vi "OpenDataLogFileForReading.vi"(0 "Filename":string) -> (1 "Data Log File Refnum":refnum<k1>, 2 "error out":errorcluster)   [LabVIEW 2010]
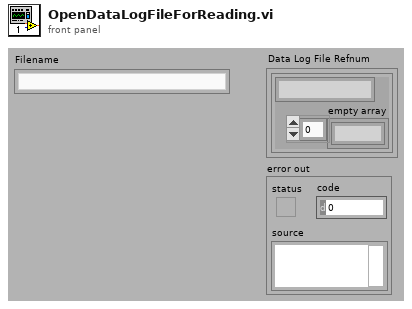
[diagram p1: front panel]
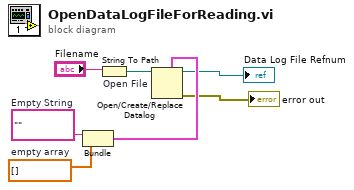
[diagram p0: block diagram]
diagram:
  w7 = ""  # Empty String
  w6 = sgl[] []  # empty array
  n1 = Bundle(w7, "empty array"=w6) -> (w3:cluster{string, "empty array":sgl[]})  [unwired: 1 out]
  n2 = String To Path(string="Filename") -> (path=w4:path)
  n3 = Open/Create/Replace Datalog "Open File"(5:w3, 11:w4) -> (0:→"error out":errorcluster, 3:→"Data Log File Refnum":refnum<k1>)  [unwired: 1 in, 4 out]
